vi "DDVL Cluster and SubPanel Refs.vi"(7 "All Objects Refs":refnum<vi>[](array[refnum])) -> (4 "Cluster Refs":refnum<vi>[](array[refnum]), 15 "Sub Panel Refs":refnum<vi>[](array[refnum]))   [LabVIEW 2016]
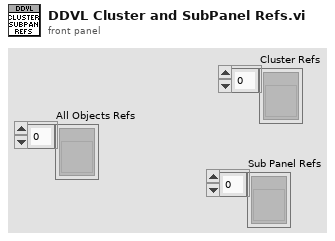
[diagram p1: front panel]
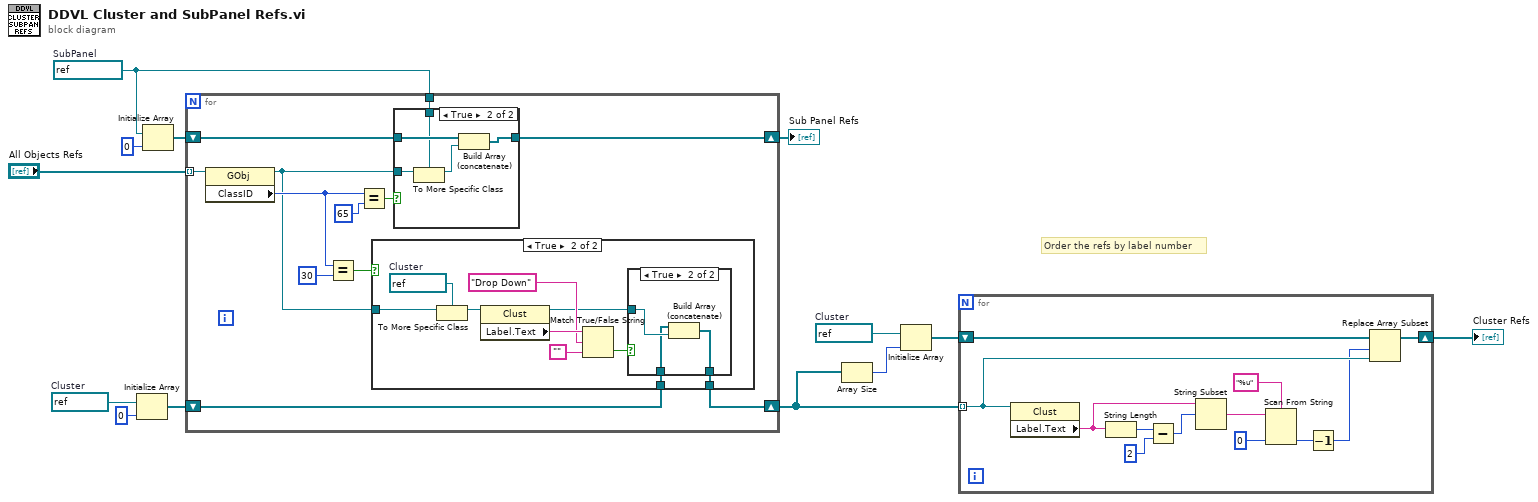
[diagram p0: block diagram]
diagram:
  w5 = refnum<vi> refnum  # Cluster
  w9 = refnum<vi> refnum  # Cluster
  w11 = refnum<vi> refnum  # SubPanel
  # "Order the refs by label number"
  n1 = Initialize Array(w9, 0 ("dimension size")) -> (w8:refnum<vi>[])
  n2 = Initialize Array(w11, 0 ("dimension size")) -> (w12:refnum<vi>[])
  n3 = for {
    tunnel: "All Objects Refs" -> [w25] mode=indexing
    shift-right: [w21] -> w7
    shift-left: w12 -> [w22]
    tunnel: w11 -> [w20]
    shift-right: [w14] -> w3
    shift-left: w8 -> [w15]
    n4 = property class="GObj"(reference=w25) -> (reference out=w16:refnum<vi>, "ClassID"=w19:u32)  [unwired: 1 in, 1 out]
    n5 = Equal?(x=w19, y=u32 30) -> (x = y?=w17:bool)
    n6 = Equal?(x=w19, y=u32 65) -> (x = y?=w23:bool)
    n7 = case shown="True" w17 {
      tunnel: w16 -> [_ w35]
      tunnel: w15 -> [w26 w29]
      tunnel: [w26 w27] -> w14
      frame False {
      }
      frame True {
        w36 = refnum<vi> refnum  # Cluster
        n8 = To More Specific Class(target class=w36, reference=w35) -> (specific class reference=w34:refnum<vi>)  [unwired: 1 in, 1 out]
        n9 = property class="Clust"(reference=w34) -> (reference out=w28:refnum<vi>, "Label.Text"=w33:string)  [unwired: 1 in, 1 out]
        n10 = Match True/False String(2:"", 3:"Drop Down" ("true string"), 4:w33) -> (0:w30:bool)  [unwired: 1 out]
        n11 = case shown="True" w30 {
          tunnel: w29 -> [w37 w39]
          tunnel: w28 -> [_ w40]
          tunnel: [w37 w38] -> w27
          frame False {
          }
          frame True {
            n12 = Build Array (concatenate)(w39, w40) -> (w38:refnum<vi>[])
          }
        }
      }
    }
    n13 = case shown="True" w23 {
      tunnel: w22 -> [w41 w46]
      tunnel: [w41 w45] -> w21
      tunnel: w16 -> [_ w44]
      tunnel: w20 -> [_ w43]
      frame False {
      }
      frame True {
        n14 = To More Specific Class(target class=w43, reference=w44) -> (specific class reference=w42:refnum<vi>)  [unwired: 1 in, 1 out]
        n15 = Build Array (concatenate)(w46, w42) -> (w45:refnum<vi>[])
      }
    }
  }
  "Sub Panel Refs" <- w7
  n16 = Array Size(array=w3) -> (size(s)=w4:i32)
  n17 = Initialize Array(w5, w4) -> (w2:refnum<vi>[])
  n18 = for {
    tunnel: w3 -> [w49] mode=indexing
    shift-right: [w48] -> w1
    shift-left: w2 -> [w51]
    n19 = property class="Clust"(reference=w49) -> ("Label.Text"=w52:string)  [unwired: 1 in, 2 out]
    n20 = String Length(string=w52) -> (length=w58:i32)
    n21 = Subtract(x=w58, y=2) -> (x-y=w56:i32)
    n22 = String Subset(string=w52, offset (0)=w56) -> (substring=w53:string)  [unwired: 1 in]
    n23 = Scan From String(format string="%u", input string=w53, default 1=0) -> (output 1=w50:i32)  [unwired: 2 in, 3 out]
    n24 = Decrement(x=w50) -> (x-1=w47:i32)
    n25 = Replace Array Subset(array=w51, new element=w49, index=w47) -> (w48:refnum<vi>[])
  }
  "Cluster Refs" <- w1
